vi "Channel Leakage Results.vi"(7 "Result":dbl=inf format="%.3g", 8 "error in":errorcluster, 9 "channel":i32=25, 10 "test case":string="PathOpen", 11 "Sequence Context":refnum<k7>) -> (0 "error out":errorcluster, 3 "Sequence Context dup":refnum<k7>)   [LabVIEW 2010]
doc: "This function transfers a single Compare Data Test (CDT) record to the current TestStand sequence step."
uses:
  Generic/TestConsole/Test Criteria Control.ctl
panel:
  in  "Acceptance Criteria":T1
  in  "Test Criteria":T1=[["TRS_tbd1", "Leakage @ 0 V", "", "-100.0", "100.0", "nA", "GELE", "%.1f", "%.1f", "0 V"], ["TRS_tbd2", "Leakage @ -20 V", "", "-5000.0", "5000.0", "nA", "GELE", "%.1f", "%.1f", "-20 V"], ["TRS_tbd3", "Leakage @ 20 V", "", "-5000.0", "5000.0", "nA", "GELE", "%.1f", "%.1f", "20 V"], ["TRS1520", "Test Set Resistance", "", "0.0", "12.0", "ohms", "GELE", "%.1f", "%.1f", "Cont"], ["", "Load Resistance", "", "494.0", "504.0", "ohms", "GELE", "%.1f", "%.1f", "Load"], ["TRS1521", "Self Test Path Open", "", "2000000", "", "ohms", "GT", "%.0f", "%.0f", "PathOpen"], ["TRS1522", "Self Test Path, Fixture Connect", "", "95000", "105000", "ohms", "GELE", "%.0f", "%.0f", "Connect"], ["TRS1523", "Self Test Path, Fixture Disconnected", "", "10000000", "", "ohms", "GT", "%.0f", "%.0f", "Disconnected"]]
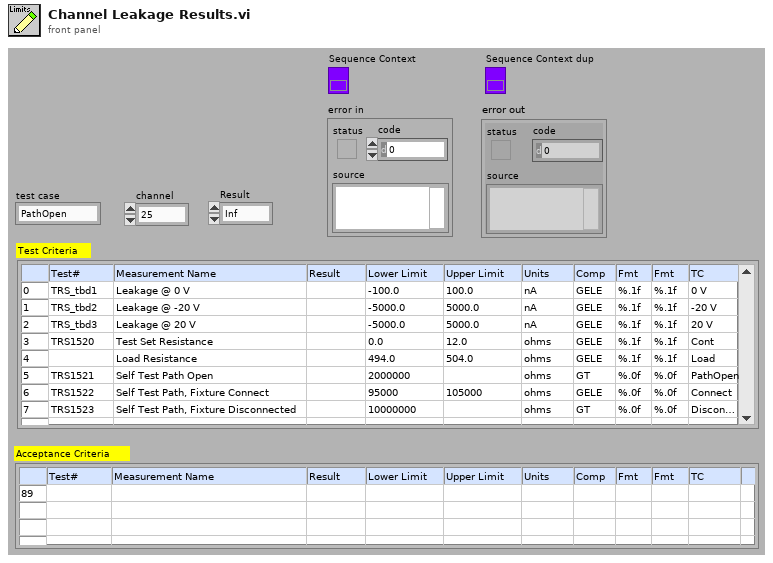
[diagram p1: front panel]
types:
  T1 = typedef "Test Criteria Control.ctl" = string[][]
  T2 = typedef "TestStand_Result Control.ctl" = cluster{"Measurement Name":string, "Result":dbl, "Low Limit":dbl, "High Limit":dbl, "Units":string, "Comp":string, "DataFmt":string, "LimitFmt":string}
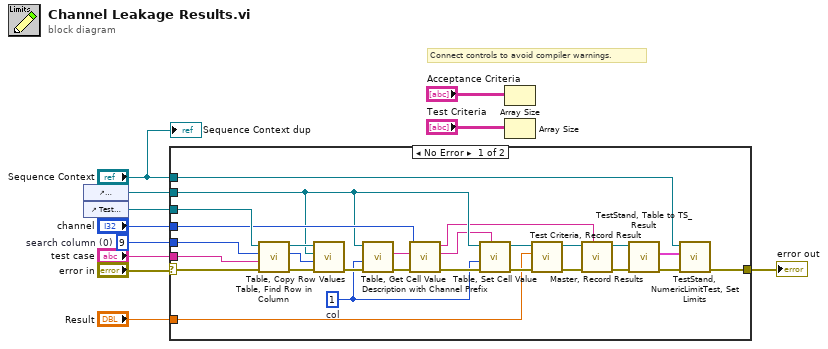
[diagram p0: block diagram]
diagram:
  w2 = 9  # search column (0)
  # "Connect controls to avoid compiler warnings."
  n1 = control-ref of="Acceptance Criteria"() -> (w4:refnum<vi>)
  n2 = control-ref of="Test Criteria"() -> (w6:refnum<vi>)
  n3 = case shown="No Error" "error in" {
    selector: "error in" -> [w13 w39]
    tunnel: [w29 w39] -> w11
    tunnel: "Sequence Context" -> [w37 _]
    tunnel: "test case" -> [w12 _]
    tunnel: w6 -> [w38 _]
    tunnel: w4 -> [w19 _]
    tunnel: "Result" -> [w30 _]
    tunnel: w2 -> [w28 _]
    tunnel: "channel" -> [w25 _]
    frame No Error {
      w15 = 1  # col
      n4 = call "Table, Find Row in Column.vi"("error in"=w13, "search key"=w12, "search column (0)"=w28, "Tbl Refnum"=w38) -> ("error out"=w35:errorcluster, "row index"=w33:i32, "Tbl Refnum out"=w34:refnum<vi>)  [unwired: 4 in, 1 out]
      n5 = call "Table, Copy Row Values.vi"("error in"=w35, "row (0)"=w33, "Tbl Refnum Dst"=w19, "Tbl Refnum Src"=w34) -> ("error out"=w21:errorcluster)  [unwired: 3 in, 2 out]
      n6 = call "Table, Get Cell Value.vi"("error in"=w21, "column (0)"=w15, "Tbl Refnum"=w19) -> ("error out"=w20:errorcluster, "cell value"=w18:string)  [unwired: 6 in, 1 out]
      n7 = call "Description with Channel Prefix.vi"("error in"=w20, "Description"=w18, "channel"=w25) -> ("error out"=w36:errorcluster, "Step Name"=w16:string, "Test Name"=w17:string)  [unwired: 4 in]
      n8 = call "Table, Set Cell Value.vi"("cell value"=w16, "error in"=w36, "column (0)"=w15, "Tbl Refnum"=w19) -> ("error out"=w32:errorcluster, "Tbl Refnum out"=w31:refnum<vi>)  [unwired: 2 in, 2 out]
      n9 = call "Test Criteria, Record Result.vi"("error in"=w32, "Result"=w30, "Tbl Refnum"=w31) -> ("error out"=w27:errorcluster, "Tbl Refnum out"=w26:refnum<vi>)  [unwired: 6 in, 1 out]
      n10 = call "Master, Record Results.vi"("step name"=w17, "error in"=w27, "Tbl Refnum"=w26) -> ("error out"=w24:errorcluster, "Tbl Refnum dup"=w22:refnum<vi>)  [unwired: 7 in]
      n11 = call "TestStand, Table to TS_Result.vi"("error in"=w24, "Tbl Refnum"=w22) -> ("error out"=w23:errorcluster, "TestStand Result"=w14:T2)  [unwired: 7 in, 1 out]
      n12 = call "TestStand, NumericLimitTest, Set Limits.vi"("error in"=w23, "CDT_type"=w14, "Sequence Context"=w37) -> ("error out"=w29:errorcluster)  [unwired: 7 in, 1 out]
    }
    frame Error {
    }
  }
  "error out" <- w11
  n13 = Array Size(array="Acceptance Criteria") -> ()  [unwired: 1 out]
  n14 = Array Size(array="Test Criteria") -> ()  [unwired: 1 out]
  "Sequence Context dup" <- "Sequence Context"
